vi "onHttpPost (File).vi"(8 "error in":errorcluster, 10 "httpRequest":refnum<class "httpRequest.lvclass">, 11 "http-method in":refnum<class "HttpClient.Basic.lvclass">) -> (0 "error out":errorcluster, 2 "httpResponse":refnum<class "httpResponse.lvclass">, 3 "http-method out":refnum<class "HttpClient.Basic.lvclass">)   [LabVIEW 2020, in "httpClient.lvlib" / "HttpClient.Basic.lvclass"]
uses:
  HttpClient.Basic.lvclass
  httpRequest/httpRequest.lvclass
  httpResponse/httpResponse.lvclass
  httpRequest/httpRequest.lvclass/httpRequest.ctl
  HttpClient.Basic.lvclass/HttpClient.Basic.ctl
  httpRequest/Read output file.vi
  httpRequest/Read url.vi
  httpRequest/Read buffer.vi
  httpRequest/Read timeout.vi
  <vilib>/httpClient/POSTFile.vi
  <vilib>/httpClient/LabVIEWHTTPClient.lvlib
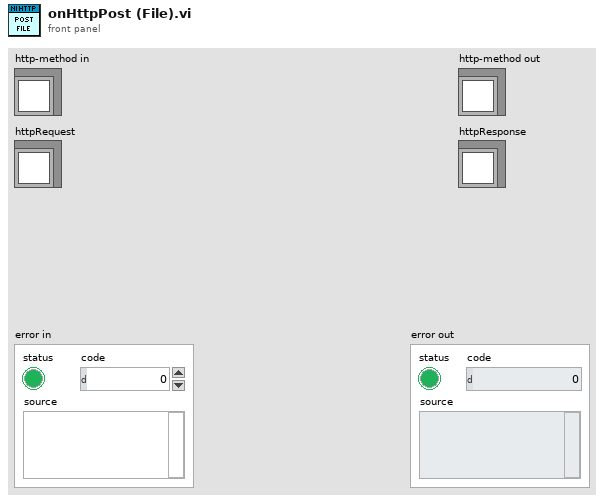
[diagram p1: front panel]
types:
  T1 = typedef "LabVIEWHTTPClient.lvlib/ClientHandle.ctl" = refnum<k1>
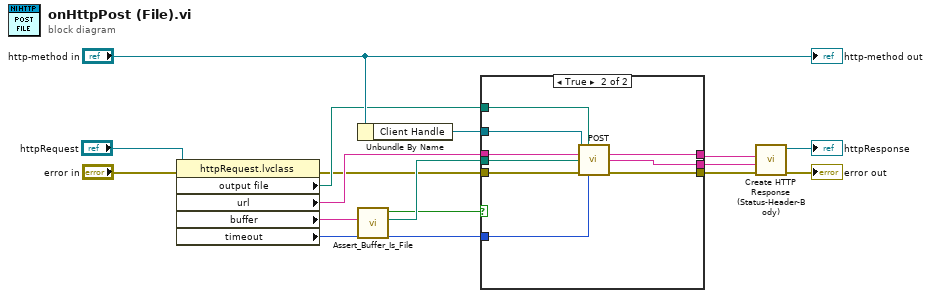
[diagram p0: block diagram]
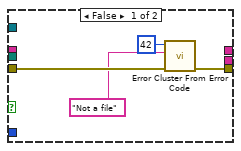
[diagram p2: hidden frame]
diagram:
  n1 = property class="httpRequest.lvclass"(reference="httpRequest", error in="error in") -> (error out=w9:errorcluster, "output file"=w11:path, "url"=w14:string, "buffer"=w13:string, "timeout"=w15:i32)  [unwired: 1 out]
  n2 = Unbundle By Name("http-method in") -> ("Client Handle"=w8:T1)
  n3 = call "Assert_Buffer_Is_File.vi"("buffer"=w13) -> ("File"=w12:path, "is File?"=w6:bool)  [unwired: 9 in]
  n4 = case shown="True" w6 {
    tunnel: [w20 w29] -> w2
    tunnel: [_ w28] -> w5
    tunnel: [_ w27] -> w4
    tunnel: w15 -> [_ w26]
    tunnel: w14 -> [_ w25]
    tunnel: w12 -> [_ w24]
    tunnel: w11 -> [_ w23]
    tunnel: w9 -> [w19 w22]
    tunnel: w8 -> [_ w21]
    frame False {
      n5 = call <vilib>:"Error Cluster From Error Code.vi"("error in (no error)"=w19, "error message (\"\")"="Not a file" ("error message (\"\")"), "error code (0)"=42) -> ("error out"=w20:errorcluster)  [unwired: 6 in]
    }
    frame True {
      n6 = call-poly <vilib>:"POST.vi"("client handle"=w21, "output file"=w23, "url"=w25, "file"=w24, "error in (no error)"=w22, "timeout (10000)"=w26) -> ("headers"=w27:string, "body"=w28:string, "error out"=w29:errorcluster)  [unwired: 6 in, 1 out]
    }
  }
  n7 = call "Create HTTP Response (Status-Header-Body).vi"("error in"=w2, "body"=w5, "Headers w/ status line(s)"=w4) -> ("error out"=→"error out":errorcluster, "httpResponse out"=→"httpResponse":refnum<class "httpResponse.lvclass">)  [unwired: 7 in]
  "http-method out" <- "http-method in"
